vi "Move Menu Up.vi"(8 "error in (no error)":errorcluster, 11 "Display State In":T1={"Numeric"=0.0, "Array of Button References"=[], "Space Between Menu Buttons"=0, "Number of Menu Buttons"=0, "Array of Button Names"=[], "Most Recent Vertical Position"=0, "This VI"=refnum, "Current Action"=enum."Not Moving", "Most Recent Distance Traveled"=0, "Method"=enum."Move Up", "Data In"=0} caption="State") -> (0 "error out":errorcluster, 3 "Display State Out":T1={"Numeric"=0.0, "Array of Button References"=[], "Space Between Menu Buttons"=0, "Number of Menu Buttons"=0, "Array of Button Names"=[], "Most Recent Vertical Position"=0, "This VI"=refnum, "Current Action"=enum."Not Moving", "Most Recent Distance Traveled"=0, "Method"=enum."Move Up", "Data In"=0} caption="State")   [LabVIEW 2011, in "Sliding Menu Library.lvlib" / "Sliding Menu XControl.xctl"]
uses:
  Sliding Menu XControl.xctl
  Sliding Menu State.ctl
  Menu Button Library/Menu Button xControl/Menu Button xControl.xctl
  Sliding Menu SubVIs/Sliding Menu Type Definitions/Current User Action.ctl
  Sliding Menu Methods.ctl
  Sliding Menu Data.ctl
  Sliding Menu Library.lvlib
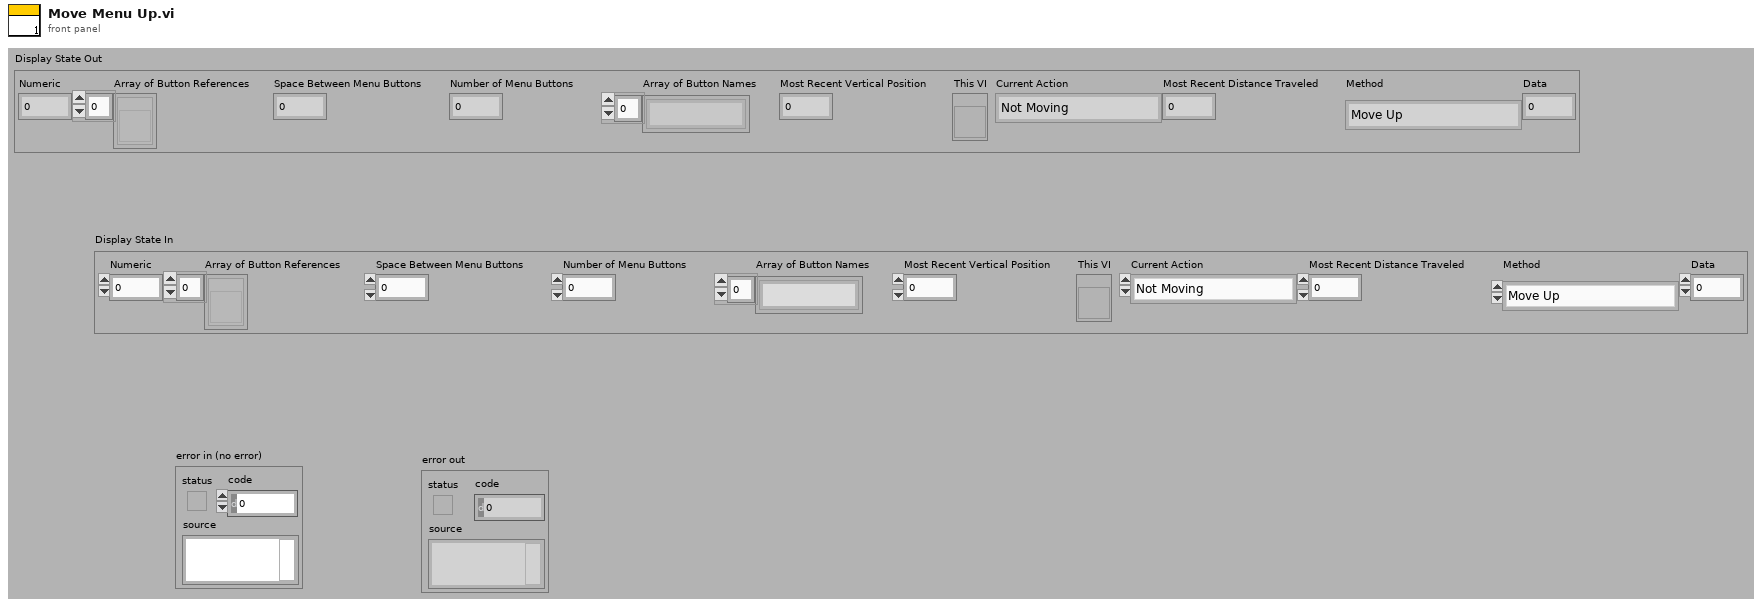
[diagram p1: front panel]
types:
  T1 = typedef "Sliding Menu Library.lvlib/Sliding Menu XControl.xctl/Sliding Menu State.ctl" = cluster{"Numeric":dbl, "Array of Button References":refnum<vi>[], "Space Between Menu Buttons":i32, "Number of Menu Buttons":i32, "Array of Button Names":string[], "Most Recent Vertical Position":i32, "This VI":refnum<vi>, "Current Action":T2, "Most Recent Distance Traveled":i32, "Method":T3, "Data In":T4}
  T2 = typedef "Sliding Menu Library.lvlib/Current User Action.ctl" = enum16{"Not Moving", "Mouse Down", "Mouse Up No Dragging", "Bounce Up Needed", "Bounce Down Needed", "Dragging", "Easing"}
  T3 = typedef "Sliding Menu Methods.ctl" = enum16{"Resize", "Move Up", "Move Down", "Move to 0"}
  T4 = typedef "Sliding Menu Library.lvlib/Sliding Menu XControl.xctl/Sliding Menu Data.ctl" = i32
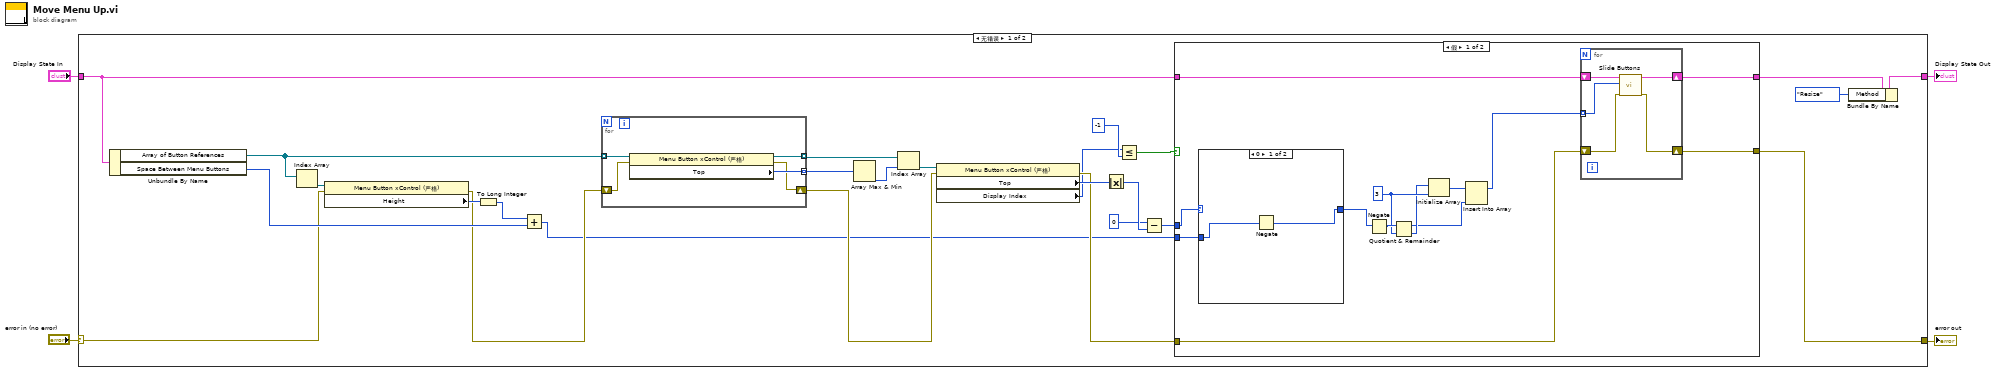
[diagram p0: block diagram]
diagram:
  n1 = case shown="无错误" "error in (no error)" {
    selector: "error in (no error)" -> [w15 w60]
    tunnel: [w11 w60] -> w1
    tunnel: "Display State In" -> [w27 w59]
    tunnel: [w29 w59] -> w2
    frame No Error {
      n2 = Unbundle By Name(w27) -> ("Array of Button References"=w23:refnum<vi>[], "Space Between Menu Buttons"=w18:i32)
      n3 = Index Array(array=w23) -> (element=w22:refnum<vi>)  [unwired: 1 in]
      n4 = property class="Menu Button xControl (严格)"(reference=w22, error in=w15) -> (error out=w14:errorcluster, "Height"=w17:u32)  [unwired: 1 out]
      n5 = To Long Integer(number=w17) -> (32bit integer=w16:i32)
      n6 = Add(x=w16, y=w18) -> (x+y=w8:i32)
      n7 = for {
        tunnel: w23 -> [w58] mode=indexing
        tunnel: [w57] -> w26 mode=indexing
        tunnel: [w56] -> w25 mode=indexing
        shift-right: [w55] -> w13
        shift-left: w14 -> [w54]
        n8 = property class="Menu Button xControl (严格)"(reference=w58, error in=w54) -> (reference out=w56:refnum<vi>, error out=w55:errorcluster, "Top"=w57:i32)
      }
      n9 = Array Max & Min(array=w26) -> (min index (indices)=w24:i32)  [unwired: 3 out]
      n10 = Index Array(array=w25, index=w24) -> (element=w21:refnum<vi>)
      n11 = property class="Menu Button xControl (严格)"(reference=w21, error in=w13) -> (error out=w12:errorcluster, "Top"=w20:i32, "Display Index"=w5:i32)  [unwired: 1 out]
      n12 = Absolute Value(x=w20) -> (abs(x)=w19:i32)
      n13 = Less Or Equal?(x=w5, y=-1 ("x")) -> (x <= y?=w6:bool)
      n14 = Subtract(x=0, y=w19) -> (x-y=w9:i32)
      n15 = case shown="假" w6 {
        tunnel: [w43 w53] -> w30
        tunnel: w27 -> [w42 w53]
        tunnel: w12 -> [w41 w52]
        tunnel: [w34 w52] -> w11
        tunnel: w9 -> [w33 _]
        tunnel: w8 -> [w31 _]
        frame False {
          w39 = 3 ("y")
          n16 = case shown="0" w33 {
            selector: w33 -> [_ w46]
            tunnel: [w44 w46] -> w32
            tunnel: w31 -> [w45 _]
            frame 0 {
              n17 = Negate(x=w45) -> (-x=w44:i32)
            }
            frame Default {
            }
          }
          n18 = Negate(x=w32) -> (-x=w40:i32)
          n19 = Quotient & Remainder(x=w40, y=w39) -> (x-y*floor(x/y)=w35:i32, floor(x/y)=w36:i32)
          n20 = Initialize Array(w36, w39) -> (w38:i32[])
          n21 = Insert Into Array(array=w38, new element=w35) -> (w37:i32[])  [unwired: 1 in]
          n22 = for {
            shift-right: [w50] -> w43
            shift-left: w42 -> [w49]
            shift-right: [w51] -> w34
            shift-left: w41 -> [w48]
            tunnel: w37 -> [w47] mode=indexing
            n23 = call "Slide Buttons.vi"("error in (no error)"=w48, "Distance"=w47, "Display State In"=w49) -> ("error out"=w51:errorcluster, "Display State Out"=w50:T1)  [unwired: 7 in]
          }
        }
        frame True {
          # "This checks to make sure you're not tyring to move lower\nthan you should"
        }
      }
      n24 = Bundle By Name(cluster=w30, "Method"=Sliding_Menu_Methods."Resize") -> (w29:T1)
    }
    frame Error {
    }
  }
  "error out" <- w1
  "Display State Out" <- w2
